vi "PomiarTESTOWYvirtual.vi"(0 "F max":dbl, 1 "ilosc probek":u32, 2 "Liniowy/Logarytmiczny":bool, 3 "Amplituda":dbl, 4 "F min":dbl, 5 "WLACZ":bool) -> (6 "V out":dbl[](array[numeric]), 7 "V in":dbl[](array[numeric]), 8 "Czestotliwosc":dbl[](array[numeric]))   [LabVIEW 2021]
uses:
  VirtualLab.lvlibp/VISASimulator/VISALib.lvlib
panel:
  out "error out 3":errorcluster
  in  "error in (no error) 2":errorcluster
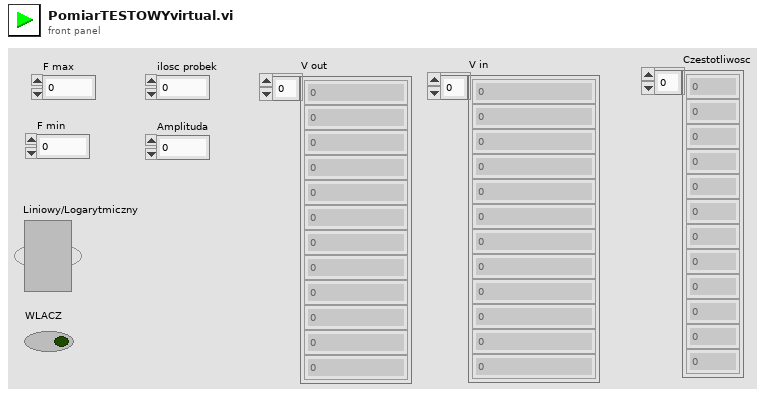
[diagram p1: front panel]
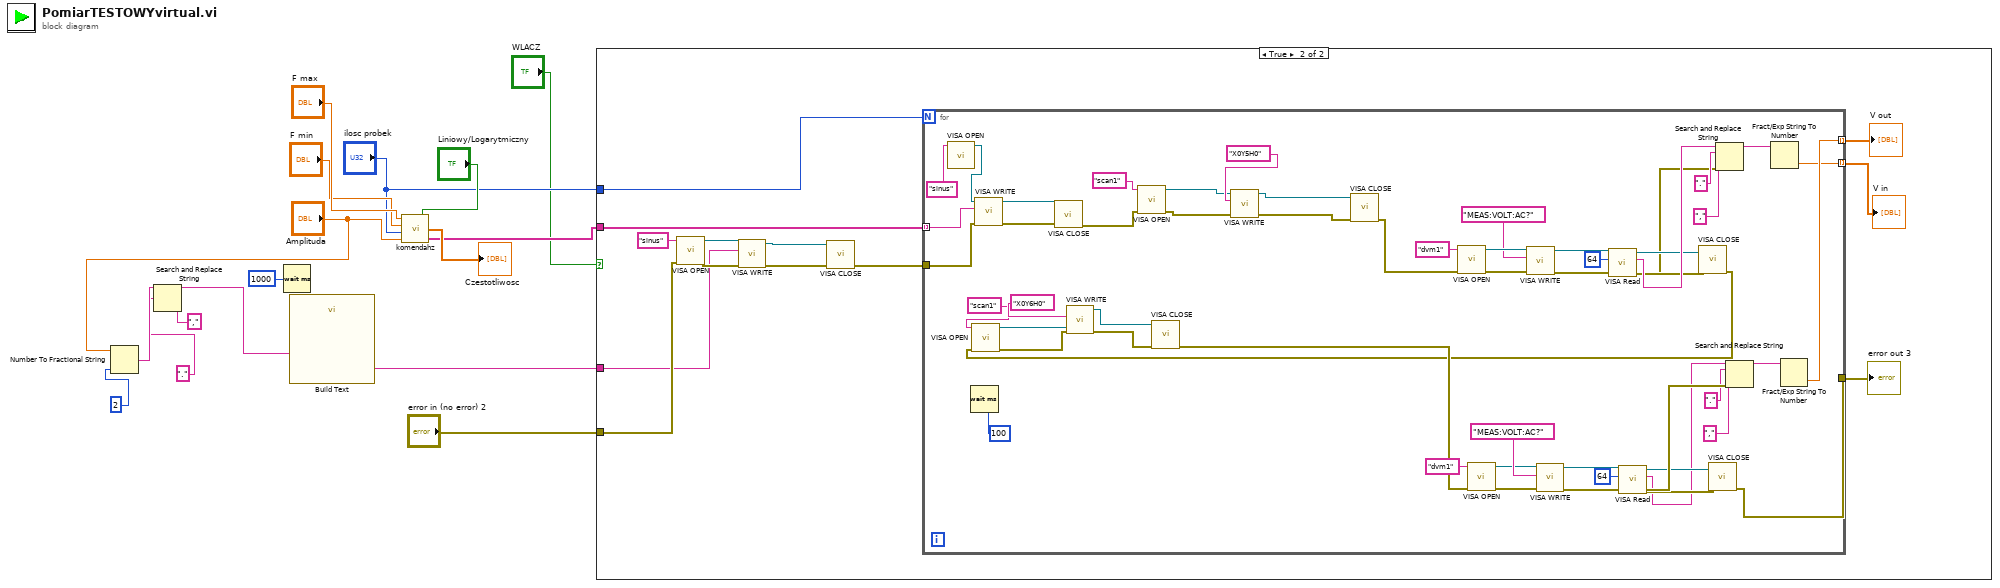
[diagram p0: block diagram]
diagram:
  n1 = Number To Fractional String(number="Amplituda", precision (6)=i16 2) -> (F-format string=w7:string)  [unwired: 2 in]
  n2 = Search and Replace String(input string=w7, search string=",", replace string="." ("replace string (\"\")")) -> (result string=w4:string)  [unwired: 5 in, 3 out]
  n3 = Wait (ms)(milliseconds to wait=u32 1000) -> ()  [unwired: 1 out]
  n4 = call "Build Text"("value"=w4) -> ("Result"=w1:string)  [unwired: 13 in, 1 out]
  n5 = call "komendahz.vi"("Liniowy/logarytmiczny"="Liniowy/Logarytmiczny", "Amplituda"="Amplituda", "ilosc probek"="ilosc probek", "F min"="F min", "F max"="F max") -> ("komendy"=w10:string[], "Czestotliwosci"=→"Czestotliwosc":dbl[])
  n6 = case shown="True" "WLACZ" {
    tunnel: "ilosc probek" -> [_ w27]
    tunnel: "error in (no error) 2" -> [_ w23]
    tunnel: w10 -> [_ w22]
    tunnel: w1 -> [_ w17]
    frame False {
    }
    frame True {
      n7 = call "VISA OPEN.vi"("error in (no error)"=w23, "VISA resource name"="sinus") -> ("error out"=w24:errorcluster, "VISA resource name out"=w28:refnum<visa-resource-name>)  [unwired: 8 in]
      n8 = call "VISA WRITE.vi"("error in (no error)"=w24, "write buffer"=w17, "VISA resource name"=w28) -> ("error out"=w25:errorcluster, "VISA resource name out"=w26:refnum<visa-resource-name>)  [unwired: 6 in, 1 out]
      n9 = call "VISA CLOSE.vi"("error in (no error)"=w25, "VISA resource name"=w26) -> ("error out"=w21:errorcluster)  [unwired: 9 in]
      n10 = for {
        N: w27 -> [_]
        tunnel: w22 -> [w81] mode=indexing
        tunnel: w21 -> [w55]
        tunnel: [w54] -> w20
        tunnel: [w50] -> w19 mode=indexing
        tunnel: [w30] -> w18 mode=indexing
        n11 = call "VISA OPEN.vi"("VISA resource name"="sinus") -> ("VISA resource name out"=w53:refnum<visa-resource-name>)  [unwired: 9 in, 1 out]
        n12 = Wait (ms)(milliseconds to wait=u32 100) -> ()  [unwired: 1 out]
        n13 = call "VISA WRITE.vi"("error in (no error)"=w55, "write buffer"=w81, "VISA resource name"=w53) -> ("error out"=w79:errorcluster, "VISA resource name out"=w80:refnum<visa-resource-name>)  [unwired: 6 in, 1 out]
        n14 = call "VISA CLOSE.vi"("error in (no error)"=w79, "VISA resource name"=w80) -> ("error out"=w72:errorcluster)  [unwired: 9 in]
        n15 = call "VISA OPEN.vi"("error in (no error)"=w72, "VISA resource name"="scan1") -> ("error out"=w48:errorcluster, "VISA resource name out"=w75:refnum<visa-resource-name>)  [unwired: 8 in]
        n16 = call "VISA WRITE.vi"("error in (no error)"=w48, "write buffer"="X0Y5H0", "VISA resource name"=w75) -> ("error out"=w46:errorcluster, "VISA resource name out"=w47:refnum<visa-resource-name>)  [unwired: 6 in, 1 out]
        n17 = call "VISA CLOSE.vi"("error in (no error)"=w46, "VISA resource name"=w47) -> ("error out"=w32:errorcluster)  [unwired: 9 in]
        n18 = call "VISA OPEN.vi"("error in (no error)"=w32, "VISA resource name"="dvm1") -> ("error out"=w41:errorcluster, "VISA resource name out"=w39:refnum<visa-resource-name>)  [unwired: 8 in]
        n19 = call "VISA WRITE.vi"("error in (no error)"=w41, "write buffer"="MEAS:VOLT:AC?", "VISA resource name"=w39) -> ("error out"=w33:errorcluster, "VISA resource name out"=w44:refnum<visa-resource-name>)  [unwired: 6 in, 1 out]
        n20 = call "VISA Read.vi"("error in (no error)"=w33, "byte count"=u32 64, "VISA resource name"=w44) -> ("error out"=w42:errorcluster, "read buffer"=w45:string, "VISA resource name out"=w40:refnum<visa-resource-name>)  [unwired: 5 in, 1 out]
        n21 = call "VISA CLOSE.vi"("error in (no error)"=w42, "VISA resource name"=w40) -> ("error out"=w31:errorcluster)  [unwired: 9 in]
        n22 = call "VISA OPEN.vi"("error in (no error)"=w31, "VISA resource name"="scan1") -> ("error out"=w71:errorcluster, "VISA resource name out"=w76:refnum<visa-resource-name>)  [unwired: 8 in]
        n23 = call "VISA WRITE.vi"("error in (no error)"=w71, "write buffer"="X0Y6H0", "VISA resource name"=w76) -> ("error out"=w58:errorcluster, "VISA resource name out"=w57:refnum<visa-resource-name>)  [unwired: 6 in, 1 out]
        n24 = call "VISA CLOSE.vi"("error in (no error)"=w58, "VISA resource name"=w57) -> ("error out"=w56:errorcluster)  [unwired: 9 in]
        n25 = call "VISA OPEN.vi"("error in (no error)"=w56, "VISA resource name"="dvm1") -> ("error out"=w61:errorcluster, "VISA resource name out"=w63:refnum<visa-resource-name>)  [unwired: 8 in]
        n26 = call "VISA WRITE.vi"("error in (no error)"=w61, "write buffer"="MEAS:VOLT:AC?", "VISA resource name"=w63) -> ("error out"=w70:errorcluster, "VISA resource name out"=w51:refnum<visa-resource-name>)  [unwired: 6 in, 1 out]
        n27 = call "VISA Read.vi"("error in (no error)"=w70, "byte count"=u32 64, "VISA resource name"=w51) -> ("error out"=w60:errorcluster, "read buffer"=w49:string, "VISA resource name out"=w62:refnum<visa-resource-name>)  [unwired: 5 in, 1 out]
        n28 = call "VISA CLOSE.vi"("error in (no error)"=w60, "VISA resource name"=w62) -> ("error out"=w54:errorcluster)  [unwired: 9 in]
        n29 = Search and Replace String(input string=w45, search string=".", replace string="," ("replace string (\"\")"), error in=w33) -> (result string=w43:string)  [unwired: 4 in, 3 out]
        n30 = Search and Replace String(input string=w49, search string=".", replace string="," ("replace string (\"\")"), error in=w70) -> (result string=w59:string)  [unwired: 4 in, 3 out]
        n31 = Fract/Exp String To Number(string=w43) -> (number=w30:dbl)  [unwired: 3 in, 1 out]
        n32 = Fract/Exp String To Number(string=w59) -> (number=w50:dbl)  [unwired: 3 in, 1 out]
      }
      "error out 3" <- w20
      "V out" <- w19
      "V in" <- w18
    }
  }
